vi "New Shortcuts.vi"(8 "error in (no error)":errorcluster) -> (0 "error out":errorcluster, 3 "StokePlotShortcuts out":refnum<class "RocketPlotShortcuts.lvclass">)   [LabVIEW 2021, in "RocketPlot.lvlib" / "RocketPlotShortcuts.lvclass"]
uses:
  RocketPlotShortcuts.lvclass
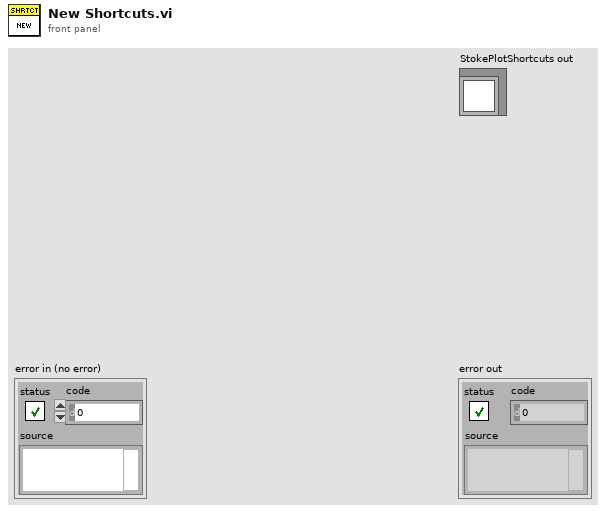
[diagram p1: front panel]
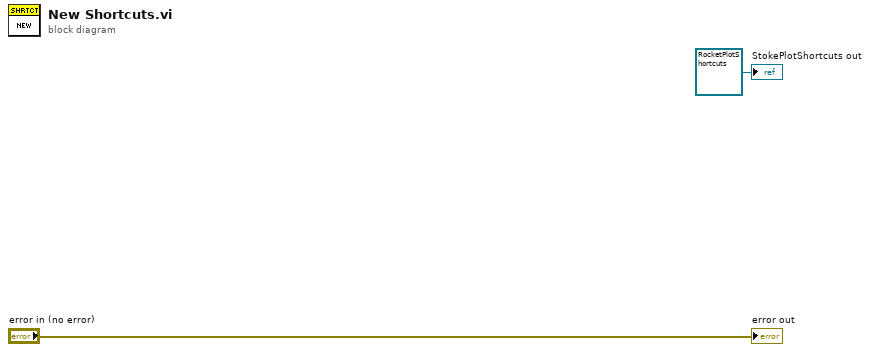
[diagram p0: block diagram]
diagram:
  "error out" <- "error in (no error)"
  "StokePlotShortcuts out" <- refnum<class "RocketPlotShortcuts.lvclass"> refnum ("StokePlotShortcuts out")
